vi "ActiveObjects_QueueQueue.vi"(7 "Action":T2=enum."GeneratePattern", 8 "error in (no error)":errorcluster, 10 "DataIn":variant, 11 "ClassRefToActOn":refnum<vi>) -> (0 "error out":errorcluster, 1 "Name":string, 2 "DataOut":variant, 3 "Cancelled":bool)   [LabVIEW 2020]
uses:
  <resource>/Framework/Providers/Open_GDS/ClassProviders/Provider_BaseClassInterface/BaseProvider_SubVIs/BaseProvider_DesignPatternsActions.ctl
  <resource>/Framework/Providers/Open_GDS/ClassProviders/Common/LvClass_class/GDSLvClass_ProviderTypes.ctl
  <resource>/Framework/Providers/Open_GDS/ClassProviders/Provider_EndevoGOOP400/EndevoG4ProviderName.ctl
  <resource>/Framework/Providers/Open_GDS/ClassProviders/Common/CommonVIs/CommonVIs_AttributeDataType.ctl
  <vilib>/picture/picture.llb/imagedata.ctl
  <resource>/Framework/Providers/Open_GDS/ClassProviders/Common/LvIcon_class/subvis/GDSLvIcon_TextDataType.ctl
  <resource>/Framework/Providers/Open_GDS/ClassProviders/Common/LvIcon_class/GDSLvIcon_WordCompressionType.ctl
  <resource>/Framework/Providers/Open_GDS/ClassProviders/Common/LvIcon_class/GDSLvIcon_TextAlignment.ctl
  <vilib>/Utility/lvfile.llb/NI_FileType.lvlib
panel:
  in  "ProcessCreation":T1(ring) caption="Process creation"
  out "NameExist1":string
  out "NameExist3":string
  out "NameExist2":string
  in  "AddInDestructor":bool
  in  "AddInConstructor":bool
  in  "StopName":string caption="Enter Stop Process Name"
  in  "StartName":string caption="Enter Start Process Name"
  in  "_Cancel":bool
  in  "_OK":bool
  in  "ProcessName":string caption="Enter Active Process Name"
  # "Active Object using Queues"
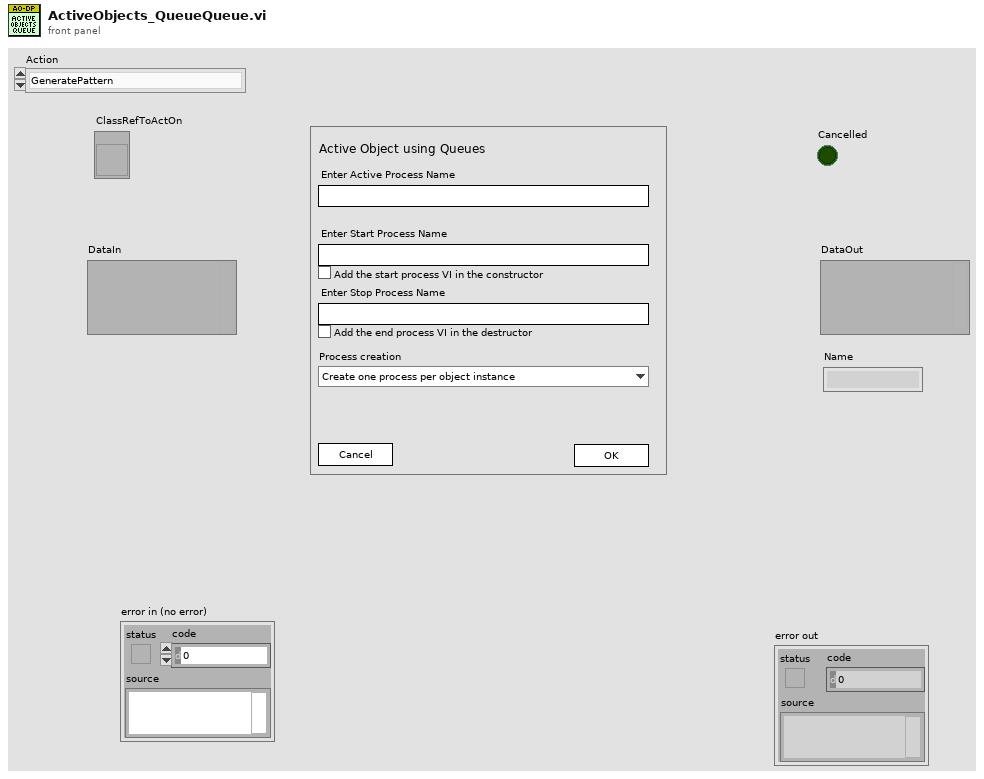
[diagram p1: front panel]
types:
  T1 = enum16{"Create one process per object instance", "Create only one process for this class"}
  T2 = typedef "BaseProvider_DesignPatternsActions.ctl" = enum16{"AddPatternDialog", "GeneratePattern", "RemovePattern", "CreatePatternMethod", "UpdatePattern"}
  T3 = typedef "GDSLvClass_ProviderTypes.ctl" = enum16{"UnKnown(LabVOOP)", "Native", "EndevoGOOP3", "OpenG(RootObject)", "OpenG(OpenG_Object)", "EndevoGOOP4", "JKI1"}
  T4 = cluster{"Data":cluster{"ProcessName":string, "StartName":string, "StopName":string, "AddInConstructor":bool, "AddInDestructor":bool, "ProcessCreation":enum16{"Create one process per object instance", "Create only one process for this class"}}, "ClassFolder":path, "SupportFolder":path, "ProcessCtl":refnum<vi>, "ProtectedFolder":refnum<vi>, "ProcessVI":refnum<vi>, "StartVI":refnum<vi>, "StopVI":refnum<vi>, "Application":refnum<vi>, "RepositoryVI":refnum<vi>, "ProcessIdRef":refnum<vi>, "ProcessRepository":path, "ClassProvider":T3, "TemplateName":string, "VI_ToFind":path, "MethodTemplate":path, "VI":refnum<vi>, "VI_ToFindSingleton":path, "Name":string}
  T5 = cluster{"ProcessName":string, "StartName":string, "StopName":string, "AddInConstructor":bool, "AddInDestructor":bool, "ProcessCreation":enum16{"Create one process per object instance", "Create only one process for this class"}}
  T6 = cluster{"Cancelled":bool, "Files":path[], "ClassPath":path, "DataOut":variant, "Name":string}
  T7 = enum8{"Enabled", "Disabled", "Disabled and Grayed Out"}
  T8 = typedef "EndevoG4ProviderName.ctl" = enum16{"EndevoGOOP400"}
  T9 = enum32{"invalid VI type", "Standard VI", "Control VI", "Global VI", "Polymorphic VI", "Configuration VI", "SubSystem", "Facade VI", "Method VI"}
  T10 = typedef "GDSLvIcon_TextDataType.ctl" = cluster{"Text":string, "Allow Only Capital Chars":bool, "Compression":T11, "Alignment":T12}
  T11 = typedef "GDSLvIcon_WordCompressionType.ctl" = enum16{"Auto", "On", "Off"}
  T12 = typedef "GDSLvIcon_TextAlignment.ctl" = enum16{"Center", "Left", "Right"}
  T13 = typedef "imagedata.ctl" = cluster{"image type":i32, "image depth":i32, "image":u8[], "mask":u8[], "colors":u32[], "Rectangle":cluster{"left":i16, "top":i16, "right":i16, "bottom":i16}}
  T14 = typedef "GDSLvCLass_ClassSettingsType.ctl" = cluster{"ClassProviderName":string, "ClassTemplateUsed":string, "ClassTemplateVersion":string, "ClassDescription":string, "PlugIns":T15[], "ConnectorPanePattern":string}
  T15 = typedef "GDSLvClass_PlugIn.ctl" = cluster{"Type":T16, "ID":string, "Version":string, "Path":path, "Name":string, "Data":variant}
  T16 = typedef "GDSLvClass_PlugInTypes.ctl" = enum16{"DesignPattern", "MethodTypes"}
  T17 = typedef "GOOP400_Options.ctl" = cluster{"FlatFolderStructure":bool}
  T18 = enum32{"invalid scope", "public", "private", "protected"}[]
  T19 = typedef "CommonVIs_AttributeDataType.ctl" = enum16{"UINT8", "INT8", "UINT16", "INT16", "UINT32", "INT32", "UINT64", "INT64", "SGL", "DBL", "EXT", "CSG", "CDB", "CXT", "TimeStamp", "STRING", "PATH", "BOOL", "ENUM", "RefNum", "VIRefNum", "LabVIEW Class", "Cluster", "Variant", "TypeDef", "Waveform", "LabVIEW Object", "Other", "void", "Set", "Map"}
  T20 = typedef "GDSLvClass_IconSettingsType.ctl" = cluster{"Frame":u32, "Frame thickness":u8, "Header Background":u32, "Header Text":u32, "ColorPublic":u32, "ColorProtected":u32, "ColorPrivate":u32, "Body Text":u32, "ClassBodyIcon":string}
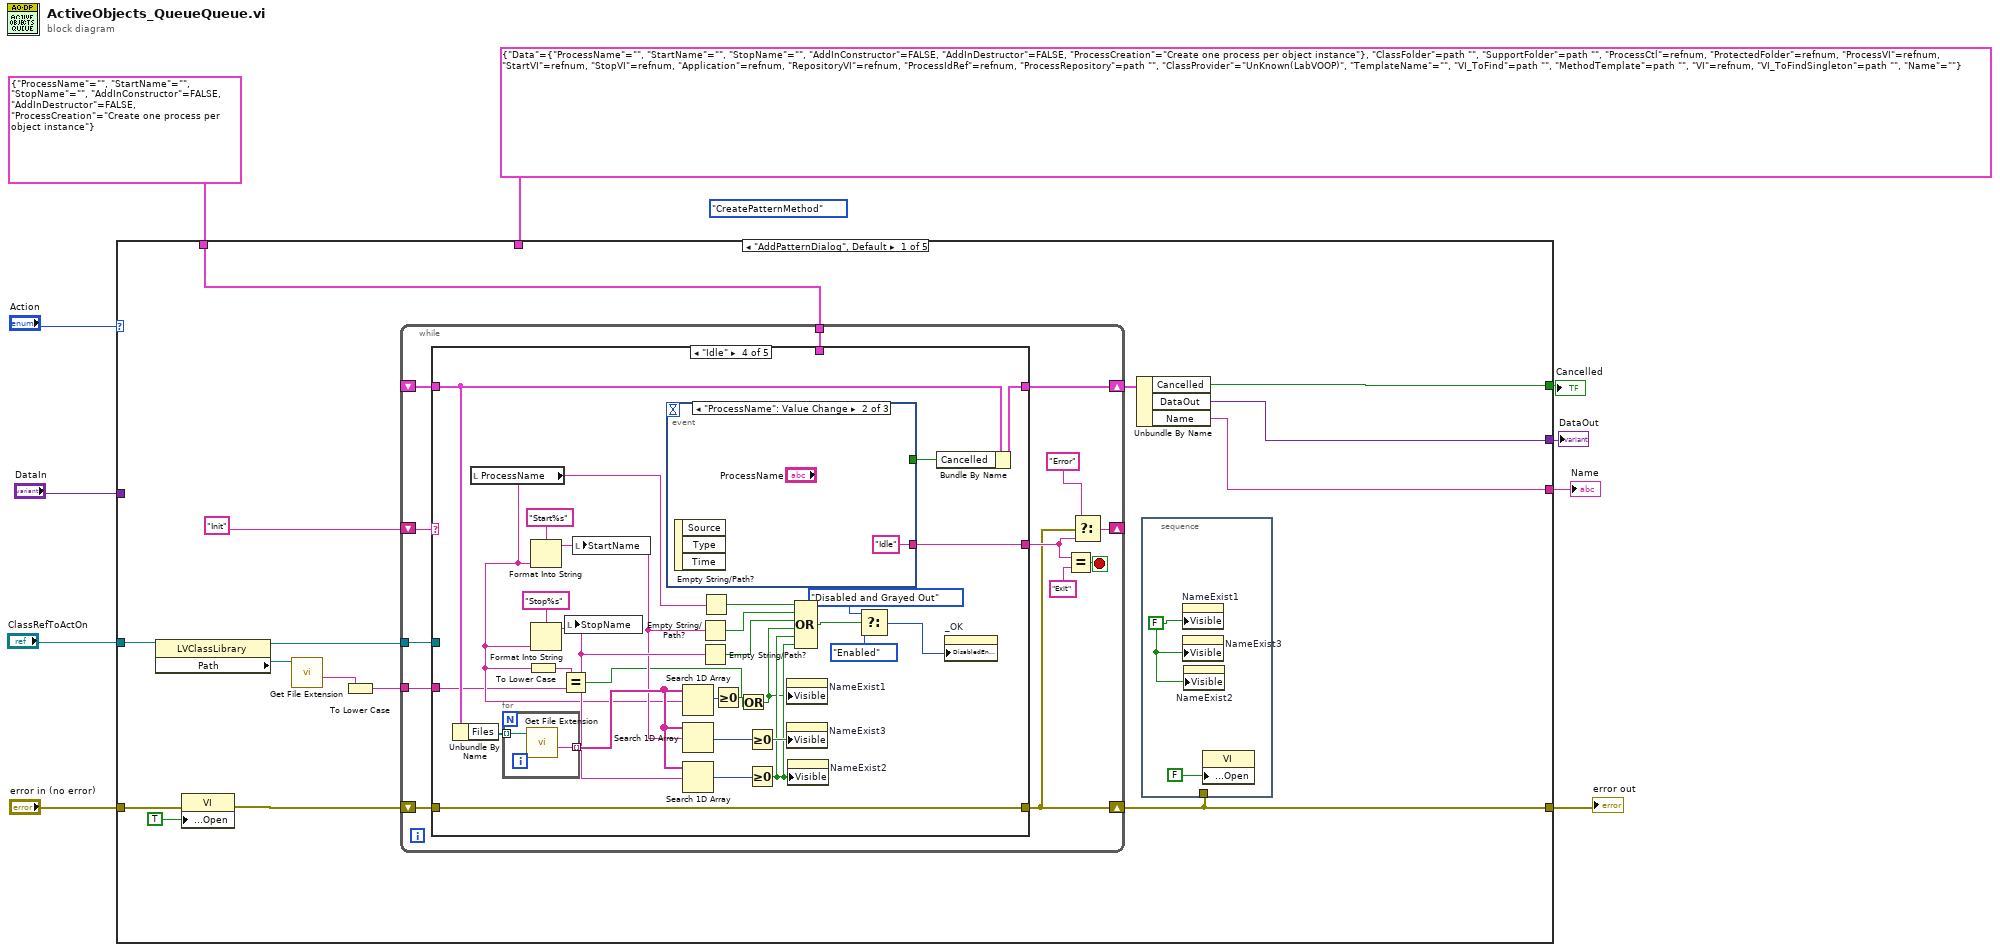
[diagram p0: block diagram]
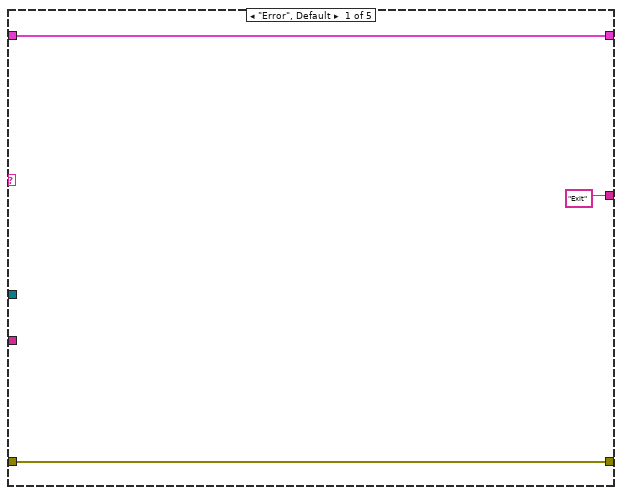
[diagram p2: hidden frame]
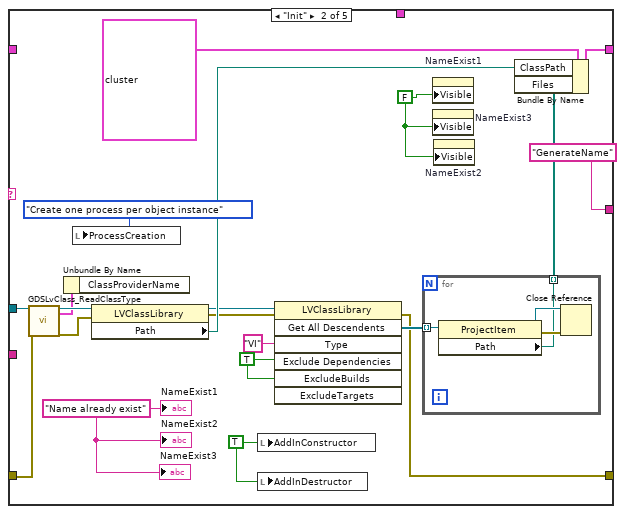
[diagram p3: hidden frame]
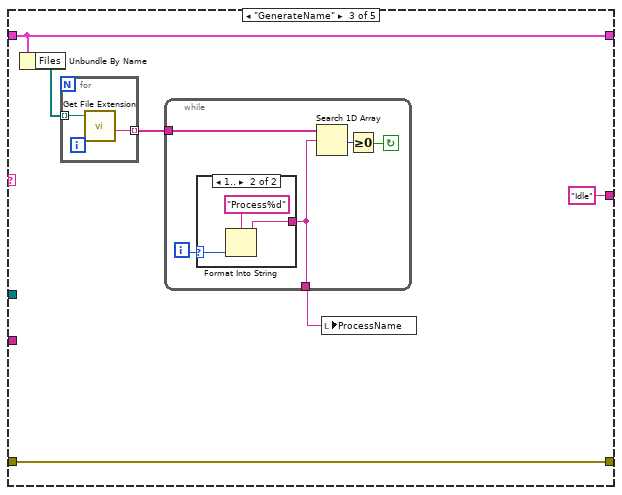
[diagram p4: hidden frame]
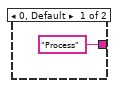
[diagram p5: hidden frame]
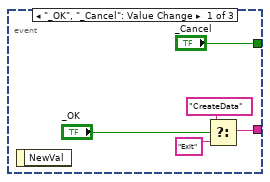
[diagram p6: hidden frame]
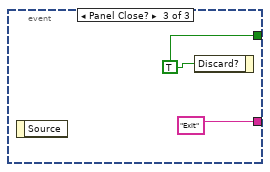
[diagram p7: hidden frame]
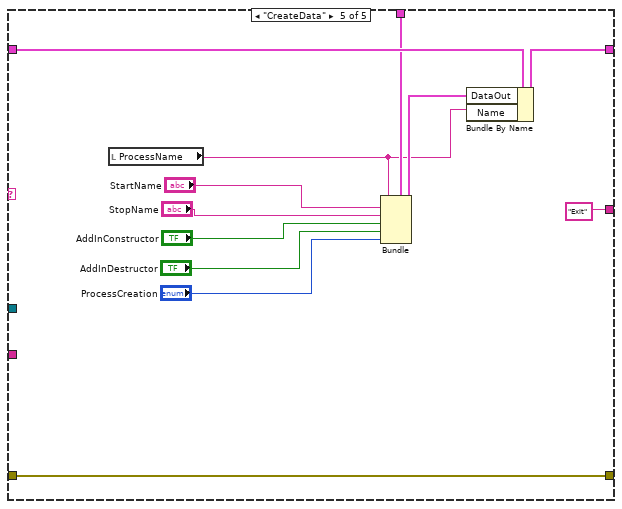
[diagram p8: hidden frame]
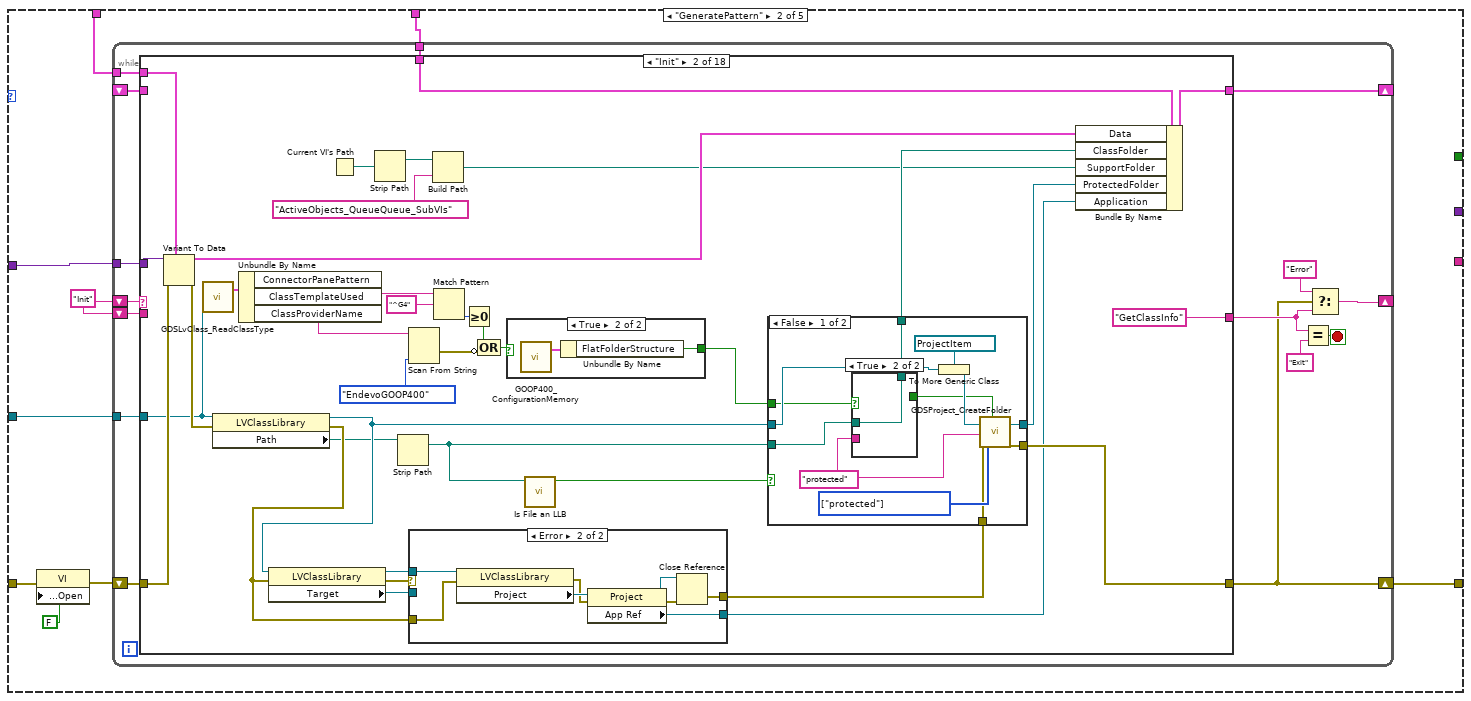
[diagram p9: hidden frame]
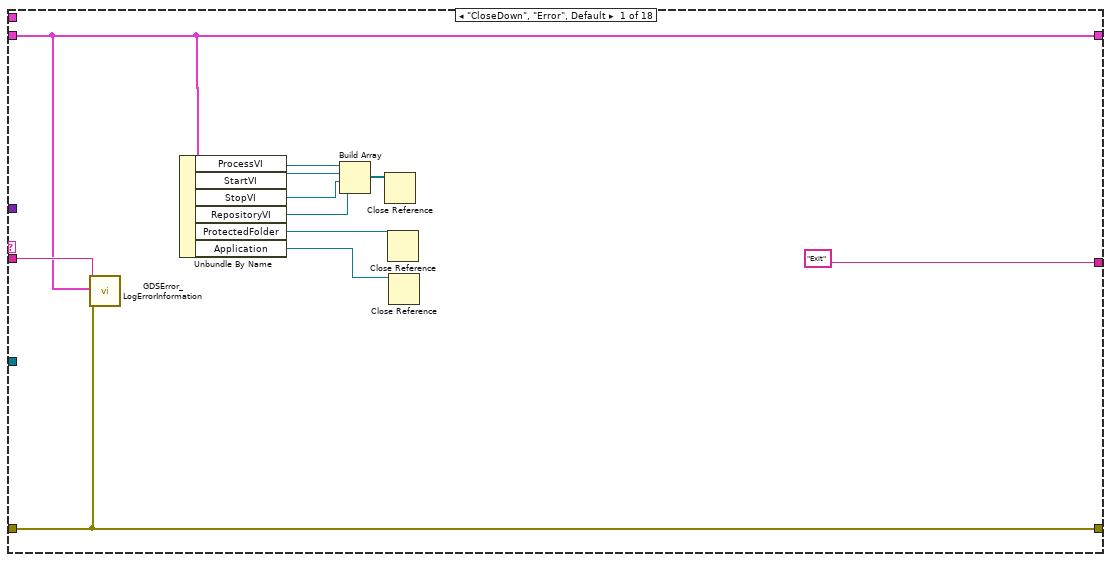
[diagram p10: hidden frame]
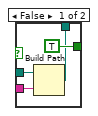
[diagram p12: hidden frame]
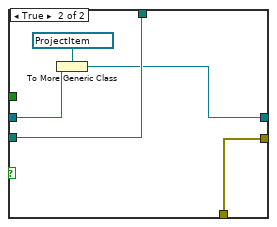
[diagram p13: hidden frame]
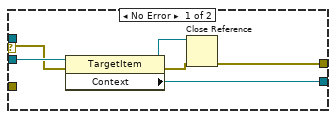
[diagram p14: hidden frame]
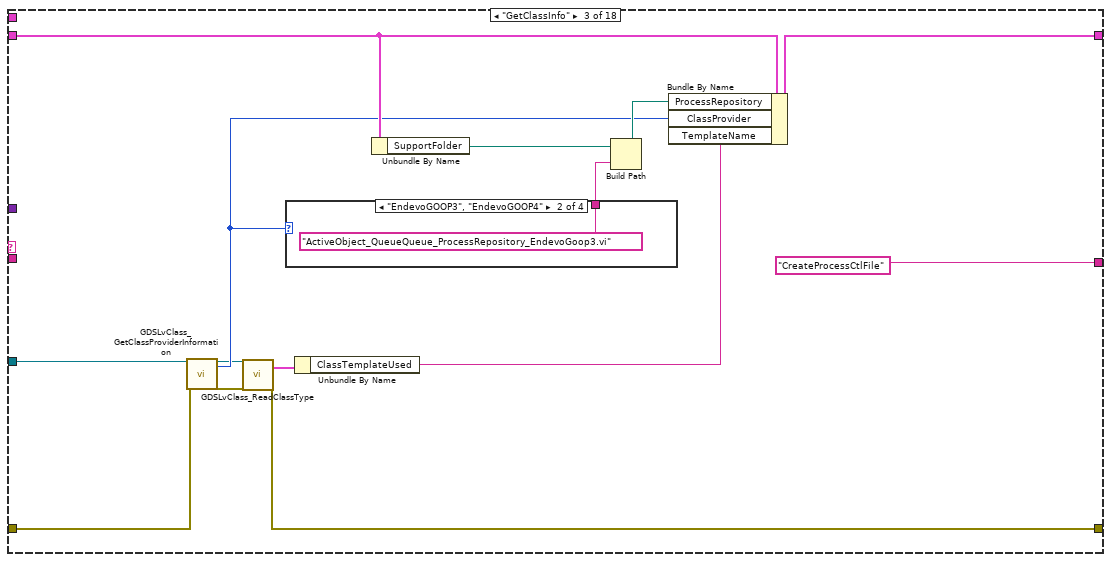
[diagram p15: hidden frame]
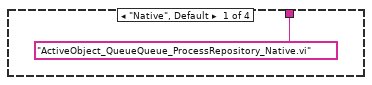
[diagram p16: hidden frame]
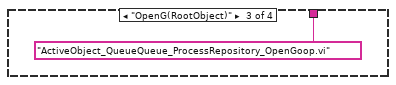
[diagram p17: hidden frame]
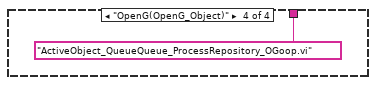
[diagram p18: hidden frame]
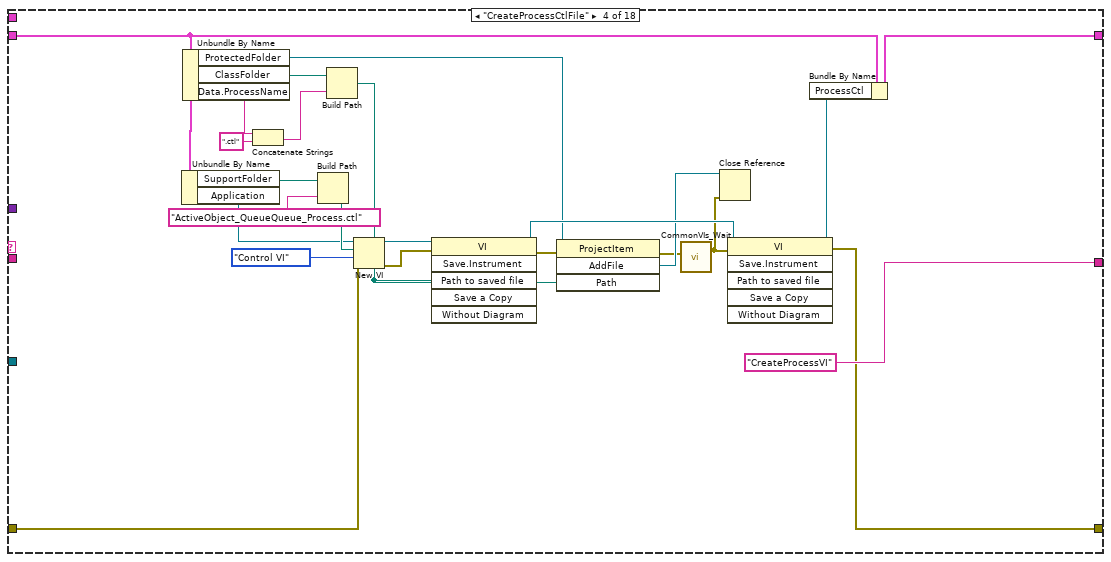
[diagram p19: hidden frame]
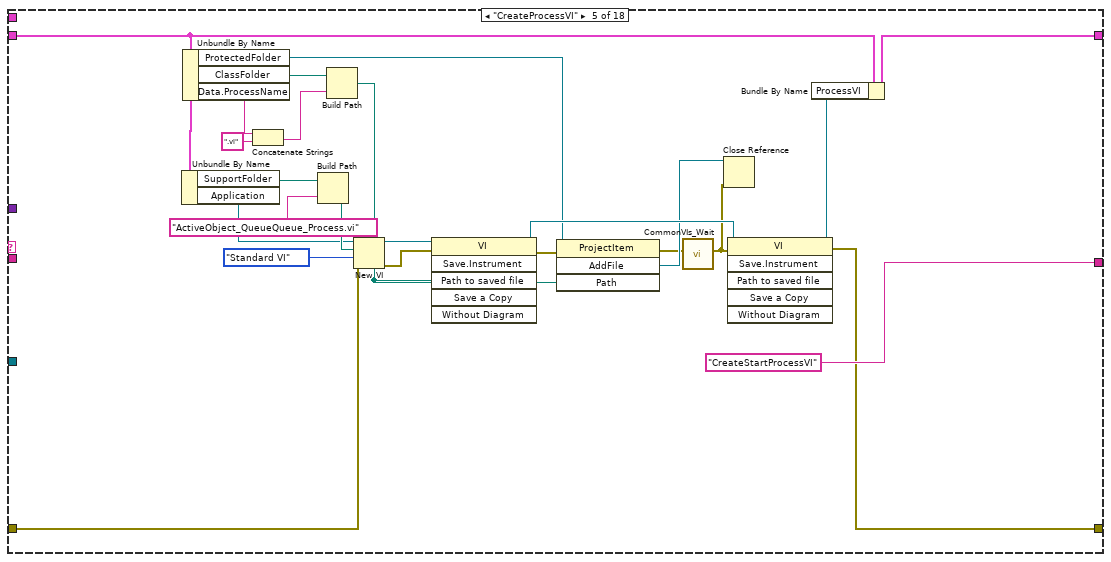
[diagram p20: hidden frame]
diagram:
  (unwired) BaseProvider_DesignPatternsActions."CreatePatternMethod" ("Action")
  n1 = case shown="\"AddPatternDialog\", Default" "Action" {
    tunnel: "error in (no error)" -> [w24 w138 w724 w725 w731]
    tunnel: [w21 w144 w724 w725 w726] -> w8
    tunnel: "ClassRefToActOn" -> [w14 w140 _ _ w730]
    tunnel: [w19 _ _ _ _] -> w6
    tunnel: [w18 _ _ _ _] -> w5
    tunnel: T5 {"ProcessName"="", "StartName"="", "StopName"="", "AddInConstructor"=FALSE, "AddInDestructor"=FALSE, "ProcessCreation"=enum."Create one process per object instance"} ("output cluster") -> [w17 w142 _ _ w727]
    tunnel: "DataIn" -> [_ w143 _ _ w729]
    tunnel: T4 {"Data"={"ProcessName"="", "StartName"="", "StopName"="", "AddInConstructor"=FALSE, "AddInDestructor"=FALSE, "ProcessCreation"=enum."Create one process per object instance"}, "ClassFolder"=path "", "SupportFolder"=path "", "ProcessCtl"=refnum, "ProtectedFolder"=refnum, "ProcessVI"=refnum, "StartVI"=refnum, "StopVI"=refnum, "Application"=refnum, "RepositoryVI"=refnum, "ProcessIdRef"=refnum, "ProcessRepository"=path "", "ClassProvider"=enum."UnKnown(LabVOOP)", "TemplateName"="", "VI_ToFind"=path "", "MethodTemplate"=path "", "VI"=refnum, "VI_ToFindSingleton"=path "", "Name"=""} -> [_ w141 _ _ w728]
    tunnel: [w16 _ _ _ _] -> w1
    frame "AddPatternDialog", Default {
      n2 = property class="LVClassLibrary"(reference=w14) -> (reference out=w13:refnum<vi>, "Path"=w15:path)  [unwired: 1 in, 1 out]
      n3 = property class="VI"(error in=w24, "Front Panel.Open"=TRUE ("Front Panel Window:Open")) -> (error out=w23:errorcluster)  [unwired: 1 in, 1 out]
      n4 = call <vilib>:"Get File Extension.vi"("file"=w15) -> ("filename without extension"=w11:string)  [unwired: 6 in, 4 out]
      n5 = To Lower Case(string=w11) -> (all lower case string=w12:string)
      n6 = while {
        shift-right: [w33] -> w21
        shift-left: w23 -> [w40]
        shift-right: [w38] -> _
        shift-left: "Init" -> [w39]
        shift-right: [w32] -> w20
        shift-left: _ -> [w31]
        tunnel: w13 -> [w30]
        tunnel: w17 -> [w29]
        tunnel: w12 -> [w28]
        stop <- w37 stop-if-true
        n7 = case shown="\"Idle\"" w39 {
          tunnel: w40 -> [w43 w47 w68 w112 w127]
          tunnel: [w43 w59 w68 w112 w127] -> w33
          tunnel: ["Exit" "GenerateName" "Idle" w113 "Exit"] -> w34
          tunnel: [w41 w57 w69 w111 w129] -> w32
          tunnel: w31 -> [w41 _ w69 w106 w131]
          tunnel: w30 -> [_ w49 _ _ _]
          tunnel: w29 -> [_ _ _ _ w126]
          tunnel: w28 -> [_ _ _ w87 _]
          frame "Error", Default {
          }
          frame "Init" {
            w50 = "Name already exist" ("NameExist1")
            w51 = FALSE ("Visible")
            w52 = TRUE ("AddInConstructor")
            w61 = TRUE ("ExcludeDependencies")
            n8 = call <resource>:"GDSLvClass_ReadClassType.vi"("Class Refnum In"=w49, "error in (no error)"=w47) -> ("Class Refnum Out"=w48:refnum<vi>, "ClassSettings"=w45:T14, "error out"=w46:errorcluster)  [unwired: 15 in]
            n9 = Unbundle By Name(w45) -> ()  [unwired: 1 out]
            n10 = local write "ProcessCreation"(T1."Create one process per object instance" ("ProcessCreation")) -> ()
            n11 = property class="LVClassLibrary"(reference=w48, error in=w46) -> (reference out=w54:refnum<vi>, error out=w53:errorcluster, "Path"=w56:path)
            n12 = local write "AddInConstructor"(w52) -> ()
            n13 = local write "AddInDestructor"(w52) -> ()
            n14 = invoke class="LVClassLibrary" method="Get All Descendents"(reference=w54, error in=w53, "Type"="VI", "Exclude Dependencies"=w61, "ExcludeBuilds"=w61) -> (error out=w59:errorcluster, "All Descendents"=w60:refnum<vi>[])  [unwired: 2 in, 5 out]
            n15 = for {
              tunnel: w60 -> [w67] mode=indexing
              tunnel: [w64] -> w55 mode=indexing
              n16 = property class="ProjectItem"(reference=w67) -> (reference out=w65:refnum<vi>, error out=w66:errorcluster, "Path"=w64:path)  [unwired: 1 in]
              n17 = Close Reference(reference=w65, error in (no error)=w66) -> ()  [unwired: 1 out]
            }
            n18 = property on="NameExist1" class="Str"("Visible"=w51) -> ()  [unwired: 2 in, 2 out]
            n19 = property on="NameExist3" class="Str"("Visible"=w51) -> ()  [unwired: 2 in, 2 out]
            n20 = property on="NameExist2" class="Str"("Visible"=w51) -> ()  [unwired: 2 in, 2 out]
            n21 = Bundle By Name(cluster=T6 {"Cancelled"=FALSE, "Files"=[], "ClassPath"=path "", "DataOut"=variant, "Name"=""}, "ClassPath"=w56, "Files"=w55) -> (w57:T6)
            "NameExist2" <- w50
            "NameExist3" <- w50
            "NameExist1" <- w50
          }
          frame "GenerateName" {
            n22 = Unbundle By Name(w69) -> ("Files"=w73:path[])
            n23 = for {
              tunnel: w73 -> [w84] mode=indexing
              tunnel: [w83] -> w72 mode=indexing
              n24 = call <vilib>:"Get File Extension.vi"("file"=w84) -> ("filename without extension"=w83:string)  [unwired: 6 in, 4 out]
            }
            n25 = while {
              tunnel: w72 -> [w77]
              tunnel: [w74] -> w71
              i -> [w78]
              stop <- w75 continue-if-true
              n26 = case shown="1.." w78 {
                selector: w78 -> [_ w81]
                tunnel: ["Process" ("format string") w80] -> w74
                frame 0, Default {
                }
                frame 1.. {
                  n27 = Format Into String(format string="Process%d", w81) -> (resulting string=w80:string)  [unwired: 2 in, 1 out]
                }
              }
              n28 = Search 1D Array(1D array=w77, element=w74) -> (index of element=w76:i32)  [unwired: 1 in]
              n29 = Greater Or Equal To 0?(x=w76) -> (x >= 0?=w75:bool)
            }
            n30 = local write "ProcessName"(w71) -> ()
          }
          frame "Idle" {
            n31 = Unbundle By Name(w106) -> ("Files"=w107:path[])
            n32 = local read "ProcessName"() -> (w88:string)
            n33 = for {
              tunnel: w107 -> [w115] mode=indexing
              tunnel: [w114] -> w105 mode=indexing
              n34 = call <vilib>:"Get File Extension.vi"("file"=w115) -> ("filename without extension"=w114:string)  [unwired: 6 in, 4 out]
            }
            n35 = To Lower Case(string=w88) -> (all lower case string=w89:string)
            n36 = Format Into String(format string="Start%s", w88) -> (resulting string=w98:string)  [unwired: 2 in, 1 out]
            n37 = Format Into String(format string="Stop%s", w88) -> (resulting string=w99:string)  [unwired: 2 in, 1 out]
            n38 = Equal?(x=w89, y=w87) -> (x = y?=w86:bool)
            n39 = local write "StopName"(w99) -> ()
            n40 = local write "StartName"(w98) -> ()
            n41 = event shown="[1] \"ProcessName\": Value Change" {
              selector: _ -> [_ _ _]
              dyn-events: _ -> [_ _ _]
              timeout: _ -> [_ _ _]
              tunnel: [w119 "Idle" "Exit"] -> w113
              tunnel: ["_Cancel" _ w122] -> w110
              event "_OK", "_Cancel": Value Change {
                n42 = event-data() -> ()  [unwired: 1 in, 1 out]
                n43 = Select(t="CreateData", s="_OK", f="Exit") -> (s? t:f=w119:string)
              }
              event "ProcessName": Value Change {
                n44 = event-data() -> ()  [unwired: 1 in, 3 out]
              }
              event Panel Close? {
                w122 = TRUE ("Discard?")
                n45 = event-data() -> ()  [unwired: 1 in, 1 out]
                n46 = event-data("Discard?"=w122) -> ()  [unwired: 1 in, 1 out]
              }
            }
            n47 = Search 1D Array(1D array=w105, element=w88) -> (index of element=w104:i32)  [unwired: 1 in]
            n48 = Search 1D Array(1D array=w105, element=w98) -> (index of element=w103:i32)  [unwired: 1 in]
            n49 = Search 1D Array(1D array=w105, element=w99) -> (index of element=w102:i32)  [unwired: 1 in]
            n50 = Empty String/Path?(string/path=w98) -> (empty?=w96:bool)
            n51 = Empty String/Path?(string/path=w99) -> (empty?=w97:bool)
            n52 = Empty String/Path?(string/path=w88) -> (empty?=w95:bool)
            n53 = Greater Or Equal To 0?(x=w104) -> (x >= 0?=w90:bool)
            n54 = Or(x=w86, y=w90) -> (x .or. y?=w85:bool)
            n55 = Greater Or Equal To 0?(x=w103) -> (x >= 0?=w101:bool)
            n56 = Greater Or Equal To 0?(x=w102) -> (x >= 0?=w100:bool)
            n57 = property on="NameExist1" class="Str"("Visible"=w85) -> ()  [unwired: 2 in, 2 out]
            n58 = property on="NameExist3" class="Str"("Visible"=w101) -> ()  [unwired: 2 in, 2 out]
            n59 = property on="NameExist2" class="Str"("Visible"=w100) -> ()  [unwired: 2 in, 2 out]
            n60 = Compound Arithmetic op=OR(w95, w96, w97, w85, w100, w100) -> (w94:bool)
            n61 = Select(t=T7."Disabled and Grayed Out" ("Disabled"), s=w94, f=T7."Enabled" ("Disabled")) -> (s? t:f=w91:T7)
            n62 = Bundle By Name(cluster=w106, "Cancelled"=w110) -> (w111:T6)
            n63 = property on="_OK" class="Bool"("DisabledEnum"=w91) -> ()  [unwired: 2 in, 2 out]
          }
          frame "CreateData" {
            n64 = local read "ProcessName"() -> (w124:string)
            n65 = Bundle(cluster=w126, "ProcessName"=w124, "StartName"="StartName", "StopName"="StopName", "AddInConstructor"="AddInConstructor", "AddInDestructor"="AddInDestructor", "ProcessCreation"="ProcessCreation") -> (w130:T5)
            n66 = Bundle By Name(cluster=w131, "DataOut"=w130, "Name"=w124) -> (w129:T6)
          }
        }
        n67 = Equal?(x=w34, y="Exit") -> (x = y?=w37:bool)
        n68 = Select(t="Error", s=w33, f=w34) -> (s? t:f=w38:string)
      }
      n69 = Unbundle By Name(w20) -> ("Cancelled"=w19:bool, "DataOut"=w18:variant, "Name"=w16:string)
      n70 = stacked-sequence {
        tunnel: w21 -> [_]
        frame #0 {
          w26 = FALSE ("Visible")
          n71 = property on="NameExist1" class="Str"("Visible"=w26) -> ()  [unwired: 2 in, 2 out]
          n72 = property on="NameExist3" class="Str"("Visible"=w26) -> ()  [unwired: 2 in, 2 out]
          n73 = property on="NameExist2" class="Str"("Visible"=w26) -> ()  [unwired: 2 in, 2 out]
          n74 = property class="VI"("Front Panel.Open"=FALSE ("Front Panel Window:Open")) -> ()  [unwired: 2 in, 2 out]
        }
      }
    }
    frame "GeneratePattern" {
      w136 = "Init"
      n75 = property class="VI"(error in=w138, "Front Panel.Open"=FALSE ("Front Panel Window:Open")) -> (error out=w137:errorcluster)  [unwired: 1 in, 1 out]
      n76 = while {
        shift-right: [w152] -> w144
        shift-left: w137 -> [w159]
        shift-right: [w157] -> _
        shift-left: w136 -> [w158]
        shift-right: [w151] -> _
        shift-left: _ -> [w150]
        tunnel: w143 -> [w149]
        tunnel: w142 -> [w148]
        tunnel: w141 -> [w147]
        tunnel: w140 -> [w146]
        shift-left: w136 -> [w145]
        stop <- w156 stop-if-true
        n77 = case shown="\"Init\"" w158 {
          tunnel: w159 -> [w162 w200 w256 w282 w306 w331 w357 w383 w399 w408 w437 w461 w484 w488 w544 w598 w651 w710]
          tunnel: [w162 w193 w247 w268 w292 w318 w344 w374 w389 w405 w420 w449 w475 w487 w543 w596 w649 w717] -> w152
          tunnel: ["Exit" "GetClassInfo" "CreateProcessCtlFile" "CreateProcessVI" "CreateStartProcessVI" "CreateStopProcessVI" "CreateProcessRepositoryVI" w367 "UpdateOORefInVIs" w404 "UpdateVIs" "UpdateRepositoryStaticVI" "FixViRefType" "UpdateIcons" "UpdateCreate?" "UpdateDestroy?" "SaveAll" "CloseDown"] -> w153
          tunnel: [w165 w205 w250 w271 w295 w321 w346 w376 w393 w412 w435 w441 w470 w489 w546 w594 w647 w712] -> w151
          tunnel: w150 -> [w165 _ w253 w272 w296 w322 w347 w365 w394 w412 w435 w441 w470 w489 w546 w594 w647 w712]
          tunnel: w149 -> [_ w204 _ _ _ _ _ _ _ _ _ _ _ _ _ _ _ _]
          tunnel: w148 -> [_ w203 _ _ _ _ _ _ _ _ _ _ _ _ _ _ _ _]
          tunnel: w147 -> [_ w202 _ _ _ _ _ _ _ _ _ _ _ _ _ _ _ _]
          tunnel: w146 -> [_ w174 w257 _ _ _ _ _ w391 w407 w426 _ _ _ w550 w593 w646 w716]
          tunnel: w145 -> [w169 _ _ _ _ _ _ _ _ _ _ _ _ _ _ _ _ _]
          frame "CloseDown", "Error", Default {
            n78 = call <resource>:"GDSError_LogErrorInformation.vi"("State"=w169, "LocalVariableData"=w165, "error in (no error)"=w162) -> ()  [unwired: 16 in, 1 out]
            n79 = Unbundle By Name(w165) -> ("ProcessVI"=w168:refnum<vi>, "StartVI"=w167:refnum<vi>, "StopVI"=w166:refnum<vi>, "RepositoryVI"=w164:refnum<vi>, "ProtectedFolder"=w161:refnum<vi>, "Application"=w160:refnum<vi>)
            n80 = Build Array(w168, w167, w166, w164) -> (w163:refnum<vi>[])
            n81 = Close Reference(reference=w163) -> ()  [unwired: 1 in, 1 out]
            n82 = Close Reference(reference=w161) -> ()  [unwired: 1 in, 1 out]
            n83 = Close Reference(reference=w160) -> ()  [unwired: 1 in, 1 out]
          }
          frame "Init" {
            n84 = Variant To Data(error in=w200, type=w203, Variant=w204) -> (data=w201:T5, error out=w194:errorcluster)
            n85 = call <resource>:"GDSLvClass_ReadClassType.vi"("Class Refnum In"=w174) -> ("ClassSettings"=w175:T14)  [unwired: 16 in, 2 out]
            n86 = property class="LVClassLibrary"(reference=w174, error in=w194) -> (reference out=w187:refnum<vi>, error out=w188:errorcluster, "Path"=w184:path)
            n87 = Unbundle By Name(w175) -> ("ClassTemplateUsed"=w173:string, "ClassProviderName"=w172:string)  [unwired: 1 out]
            n88 = property class="LVClassLibrary"(reference=w187, error in=w188) -> (reference out=w191:refnum<vi>, error out=w189:errorcluster, "Target"=w190:refnum<vi>)
            n89 = Current VI's Path() -> (path=w198:path)
            n90 = Strip Path(path=w198) -> (stripped path=w197:path)  [unwired: 1 out]
            n91 = Strip Path(path=w184) -> (stripped path=w182:path)  [unwired: 1 out]
            n92 = Scan From String(input string=w172, default 1=EndevoG4ProviderName."EndevoGOOP400" ("ProviderName")) -> (error out=w178:errorcluster)  [unwired: 4 in, 2 out]
            n93 = case shown="Error" w189 {
              selector: w189 -> [w232 _]
              tunnel: w190 -> [w236 _]
              tunnel: [w235 w238] -> w186
              tunnel: [w231 w239] -> w185
              tunnel: w191 -> [_ w244]
              tunnel: w188 -> [_ w243]
              frame No Error {
                n94 = property class="TargetItem"(reference=w236, error in=w232) -> (reference out=w233:refnum<vi>, error out=w234:errorcluster, "Context"=w235:refnum<vi>)
                n95 = Close Reference(reference=w233, error in (no error)=w234) -> (error out=w231:errorcluster)
              }
              frame Error {
                n96 = property class="LVClassLibrary"(reference=w244, error in=w243) -> (error out=w237:errorcluster, "Project"=w242:refnum<vi>)  [unwired: 1 out]
                n97 = property class="Project"(reference=w242, error in=w237) -> (reference out=w240:refnum<vi>, error out=w241:errorcluster, "App Ref"=w238:refnum<vi>)
                n98 = Close Reference(reference=w240, error in (no error)=w241) -> (error out=w239:errorcluster)
              }
            }
            n99 = Build Path(base path=w197, name or relative path="ActiveObjects_QueueQueue_SubVIs") -> (appended path=w195:path)
            n100 = Match Pattern(string=w173, regular expression="^G4") -> (offset past match=w179:i32)  [unwired: 1 in, 3 out]
            n101 = Greater Or Equal To 0?(x=w179) -> (x >= 0?=w177:bool)
            n102 = Compound Arithmetic op=OR(w177, invert w178) -> (w176:bool)
            n103 = case shown="True" w176 {
              tunnel: [_ w207] -> w171
              frame False {
              }
              frame True {
                n104 = call <resource>:"GOOP400_ConfigurationMemory.vi"() -> ("OptionsOut"=w208:T17)  [unwired: 18 in, 1 out]
                n105 = Unbundle By Name(w208) -> ("FlatFolderStructure"=w207:bool)
              }
            }
            n106 = call <vilib>:"Is File an LLB.vi"("path"=w182) -> ("Is LLB?"=w183:bool)  [unwired: 9 in, 1 out]
            n107 = case shown="False" w183 {
              tunnel: [w215 w227] -> w199
              tunnel: [w214 w228] -> w193
              tunnel: [w213 w226] -> w192
              tunnel: w187 -> [w212 w229]
              tunnel: w185 -> [w211 w228]
              tunnel: w182 -> [w210 w227]
              tunnel: w171 -> [w209 _]
              frame False {
                w218 = T18 [enum."protected"] items=["invalid scope", "public", "private", "protected"] ("FolderScope")
                w217 = "protected" ("name or relative path")
                n108 = case shown="True" w209 {
                  tunnel: w217 -> [w224 _]
                  tunnel: [TRUE ("CreateThePhysicalFolderIfPossible(False)") _] -> w216
                  tunnel: [w222 w225] -> w215
                  tunnel: w210 -> [w221 w225]
                  frame False {
                    n109 = Build Path(base path=w221, name or relative path=w224) -> (appended path=w222:path)
                  }
                  frame True {
                  }
                }
                n110 = To More Generic Class(target class=refnum<vi> refnum ("AddItem"), reference=w212) -> (generic class reference=w219:refnum<vi>)
                n111 = call <resource>:"GDSProject_CreateFolder.vi"("Project Item To Create Folder Below(Use MyComputer if not wired)"=w219, "FolderName"=w217, "error in (no error)"=w211, "FolderScope"=w218, "CreateThePhysicalFolderIfPossible(False)"=w216) -> ("ItemOut"=w213:refnum<vi>, "error out"=w214:errorcluster)  [unwired: 11 in, 2 out]
              }
              frame True {
                n112 = To More Generic Class(target class=refnum<vi> refnum ("AddItem"), reference=w229) -> (generic class reference=w226:refnum<vi>)
              }
            }
            n113 = Bundle By Name(cluster=w202, "Data"=w201, "ClassFolder"=w199, "SupportFolder"=w195, "ProtectedFolder"=w192, "Application"=w186) -> (w205:T4)
          }
          frame "GetClassInfo" {
            n114 = call <resource>:"GDSLvClass_GetClassProviderInformation.vi"("Class Refnum In"=w257, "error in (no error)"=w256) -> ("Class Refnum Out"=w249:refnum<vi>, "ClassProvider"=w251:T3, "error out"=w248:errorcluster)  [unwired: 15 in]
            n115 = call <resource>:"GDSLvClass_ReadClassType.vi"("Class Refnum In"=w249, "error in (no error)"=w248) -> ("ClassSettings"=w246:T14, "error out"=w247:errorcluster)  [unwired: 15 in, 1 out]
            n116 = case shown="\"EndevoGOOP3\", \"EndevoGOOP4\"" w251 {
              tunnel: ["ActiveObject_QueueQueue_ProcessRepository_Native.vi" ("name or relative path") "ActiveObject_QueueQueue_ProcessRepository_EndevoGoop3.vi" ("name or relative path") "ActiveObject_QueueQueue_ProcessRepository_OpenGoop.vi" ("name or relative path") "ActiveObject_QueueQueue_ProcessRepository_OGoop.vi" ("name or relative path")] -> w254
              frame "Native", Default {
              }
              frame "EndevoGOOP3", "EndevoGOOP4" {
              }
              frame "OpenG(RootObject)" {
              }
              frame "OpenG(OpenG_Object)" {
              }
            }
            n117 = Unbundle By Name(w246) -> ("ClassTemplateUsed"=w245:string)
            n118 = Unbundle By Name(w253) -> ("SupportFolder"=w255:path)
            n119 = Build Path(base path=w255, name or relative path=w254) -> (appended path=w252:path)
            n120 = Bundle By Name(cluster=w253, "ProcessRepository"=w252, "ClassProvider"=w251, "TemplateName"=w245) -> (w250:T4)
          }
          frame "CreateProcessCtlFile" {
            n121 = Unbundle By Name(w272) -> ("SupportFolder"=w278:path, "Application"=w266:refnum<vi>)
            n122 = Unbundle By Name(w272) -> ("ProtectedFolder"=w267:refnum<vi>, "ClassFolder"=w286:path, "Data.ProcessName"=w285:string)
            n123 = Concatenate Strings(w285, ".ctl" ("string")) -> (w283:string)
            n124 = Build Path(base path=w278, name or relative path="ActiveObject_QueueQueue_Process.ctl") -> (appended path=w276:path)
            n125 = Build Path(base path=w286, name or relative path=w283) -> (appended path=w274:path)
            n126 = New VI(8:w282, 9:T9."Control VI" ("vi type (standard vi)"), 10:w276, 11:w266) -> (0:w279:errorcluster, 3:w280:refnum<vi>)  [unwired: 3 in]
            n127 = invoke class="VI" method="Save.Instrument"(reference=w280, error in=w279, "Path to saved file"=w274) -> (reference out=w273:refnum<vi>, error out=w275:errorcluster)  [unwired: 3 in, 4 out]
            n128 = invoke class="ProjectItem" method="AddFile"(reference=w267, error in=w275, "Path"=w274) -> (error out=w264:errorcluster, "AddFile"=w265:refnum<vi>)  [unwired: 1 in, 2 out]
            n129 = call <resource>:"CommonVIs_Wait.vi"("error in"=w264) -> ("error out"=w263:errorcluster)  [unwired: 9 in]
            n130 = Close Reference(reference=w265, error in (no error)=w263) -> ()  [unwired: 1 out]
            n131 = invoke class="VI" method="Save.Instrument"(reference=w273, error in=w263) -> (reference out=w270:refnum<vi>, error out=w268:errorcluster)  [unwired: 4 in, 4 out]
            n132 = Bundle By Name(cluster=w272, "ProcessCtl"=w270) -> (w271:T4)
          }
          frame "CreateProcessVI" {
            n133 = Unbundle By Name(w296) -> ("SupportFolder"=w302:path, "Application"=w290:refnum<vi>)
            n134 = Unbundle By Name(w296) -> ("ProtectedFolder"=w291:refnum<vi>, "ClassFolder"=w310:path, "Data.ProcessName"=w309:string)
            n135 = Concatenate Strings(w309, ".vi" ("string")) -> (w307:string)
            n136 = Build Path(base path=w302, name or relative path="ActiveObject_QueueQueue_Process.vi") -> (appended path=w300:path)
            n137 = Build Path(base path=w310, name or relative path=w307) -> (appended path=w298:path)
            n138 = New VI(8:w306, 9:T9."Standard VI" ("vi type (standard vi)"), 10:w300, 11:w290) -> (0:w303:errorcluster, 3:w304:refnum<vi>)  [unwired: 3 in]
            n139 = invoke class="VI" method="Save.Instrument"(reference=w304, error in=w303, "Path to saved file"=w298) -> (reference out=w297:refnum<vi>, error out=w299:errorcluster)  [unwired: 3 in, 4 out]
            n140 = invoke class="ProjectItem" method="AddFile"(reference=w291, error in=w299, "Path"=w298) -> (error out=w288:errorcluster, "AddFile"=w289:refnum<vi>)  [unwired: 1 in, 2 out]
            n141 = call <resource>:"CommonVIs_Wait.vi"("error in"=w288) -> ("error out"=w287:errorcluster)  [unwired: 9 in]
            n142 = Close Reference(reference=w289, error in (no error)=w287) -> ()  [unwired: 1 out]
            n143 = invoke class="VI" method="Save.Instrument"(reference=w297, error in=w287) -> (reference out=w294:refnum<vi>, error out=w292:errorcluster)  [unwired: 4 in, 4 out]
            n144 = Bundle By Name(cluster=w296, "ProcessVI"=w294) -> (w295:T4)
          }
          frame "CreateStartProcessVI" {
            n145 = Unbundle By Name(w322) -> ("SupportFolder"=w327:path, "Application"=w316:refnum<vi>, "Data.ProcessCreation"=w315:T1)
            n146 = Unbundle By Name(w322) -> ("ProtectedFolder"=w317:refnum<vi>, "ClassFolder"=w335:path, "Data.StartName"=w334:string)
            n147 = case shown="\"Create one process per object instance\", Default" w315 {
              tunnel: ["ActiveObject_QueueQueue_StartProcess_OnePerObject.vi" ("name or relative path") "ActiveObject_QueueQueue_StartProcess_OnePerClass.vi" ("name or relative path")] -> w314
              frame "Create one process per object instance", Default {
              }
              frame "Create only one process for this class" {
              }
            }
            n148 = Concatenate Strings(w334, ".vi" ("string")) -> (w332:string)
            n149 = Build Path(base path=w327, name or relative path=w314) -> (appended path=w326:path)
            n150 = Build Path(base path=w335, name or relative path=w332) -> (appended path=w324:path)
            n151 = New VI(8:w331, 9:T9."Standard VI" ("vi type (standard vi)"), 10:w326, 11:w316) -> (0:w328:errorcluster, 3:w329:refnum<vi>)  [unwired: 3 in]
            n152 = invoke class="VI" method="Save.Instrument"(reference=w329, error in=w328, "Path to saved file"=w324) -> (reference out=w323:refnum<vi>, error out=w325:errorcluster)  [unwired: 3 in, 4 out]
            n153 = invoke class="ProjectItem" method="AddFile"(reference=w317, error in=w325, "Path"=w324) -> (error out=w312:errorcluster, "AddFile"=w313:refnum<vi>)  [unwired: 1 in, 2 out]
            n154 = call <resource>:"CommonVIs_Wait.vi"("error in"=w312) -> ("error out"=w311:errorcluster)  [unwired: 9 in]
            n155 = Close Reference(reference=w313, error in (no error)=w311) -> ()  [unwired: 1 out]
            n156 = invoke class="VI" method="Save.Instrument"(reference=w323, error in=w311) -> (reference out=w320:refnum<vi>, error out=w318:errorcluster)  [unwired: 4 in, 4 out]
            n157 = Bundle By Name(cluster=w322, "StartVI"=w320) -> (w321:T4)
          }
          frame "CreateStopProcessVI" {
            n158 = Unbundle By Name(w347) -> ("SupportFolder"=w353:path, "Application"=w342:refnum<vi>)
            n159 = Unbundle By Name(w347) -> ("ProtectedFolder"=w343:refnum<vi>, "ClassFolder"=w361:path, "Data.StopName"=w360:string)
            n160 = Concatenate Strings(w360, ".vi" ("string")) -> (w358:string)
            n161 = Build Path(base path=w353, name or relative path="ActiveObject_QueueQueue_StopProcess.vi") -> (appended path=w351:path)
            n162 = Build Path(base path=w361, name or relative path=w358) -> (appended path=w349:path)
            n163 = New VI(8:w357, 9:T9."Standard VI" ("vi type (standard vi)"), 10:w351, 11:w342) -> (0:w354:errorcluster, 3:w355:refnum<vi>)  [unwired: 3 in]
            n164 = invoke class="VI" method="Save.Instrument"(reference=w355, error in=w354, "Path to saved file"=w349) -> (reference out=w348:refnum<vi>, error out=w350:errorcluster)  [unwired: 3 in, 4 out]
            n165 = invoke class="ProjectItem" method="AddFile"(reference=w343, error in=w350, "Path"=w349) -> (error out=w339:errorcluster, "AddFile"=w340:refnum<vi>)  [unwired: 1 in, 2 out]
            n166 = call <resource>:"CommonVIs_Wait.vi"("error in"=w339) -> ("error out"=w338:errorcluster)  [unwired: 9 in]
            n167 = Close Reference(reference=w340, error in (no error)=w338) -> ()  [unwired: 1 out]
            n168 = invoke class="VI" method="Save.Instrument"(reference=w348, error in=w338) -> (reference out=w345:refnum<vi>, error out=w344:errorcluster)  [unwired: 4 in, 4 out]
            n169 = Bundle By Name(cluster=w347, "StopVI"=w345) -> (w346:T4)
          }
          frame "CreateProcessRepositoryVI" {
            n170 = Unbundle By Name(w365) -> ("ClassProvider"=w364:T3)
            n171 = Unbundle By Name(w365) -> ("ProcessRepository"=w366:path, "Application"=w372:refnum<vi>)
            n172 = Unbundle By Name(w365) -> ("ProtectedFolder"=w373:refnum<vi>, "ClassFolder"=w384:path, "Data.ProcessName"=w371:string)
            n173 = Format Into String(format string="%sRepository.vi", w371) -> (resulting string=w369:string)  [unwired: 2 in, 1 out]
            n174 = New VI(8:w383, 9:T9."Standard VI" ("vi type (standard vi)"), 10:w366, 11:w372) -> (0:w380:errorcluster, 3:w381:refnum<vi>)  [unwired: 3 in]
            n175 = Build Path(base path=w384, name or relative path=w369) -> (appended path=w378:path)
            n176 = invoke class="VI" method="Save.Instrument"(reference=w381, error in=w380, "Path to saved file"=w378) -> (reference out=w377:refnum<vi>, error out=w379:errorcluster)  [unwired: 3 in, 4 out]
            n177 = invoke class="ProjectItem" method="AddFile"(reference=w373, error in=w379, "Path"=w378) -> (error out=w363:errorcluster, "AddFile"=w368:refnum<vi>)  [unwired: 1 in, 2 out]
            n178 = case shown="Default" w364 {
              tunnel: ["UpdateOORefInVIs" "AddCtlToAttribute"] -> w367
              frame Default {
              }
              frame "UnKnown(LabVOOP)", "Native" {
              }
            }
            n179 = call <resource>:"CommonVIs_Wait.vi"("error in"=w363) -> ("error out"=w362:errorcluster)  [unwired: 9 in]
            n180 = Close Reference(reference=w368, error in (no error)=w362) -> ()  [unwired: 1 out]
            n181 = invoke class="VI" method="Save.Instrument"(reference=w377, error in=w362) -> (reference out=w375:refnum<vi>, error out=w374:errorcluster)  [unwired: 4 in, 4 out]
            n182 = Bundle By Name(cluster=w365, "RepositoryVI"=w375) -> (w376:T4)
          }
          frame "AddCtlToAttribute" {
            w387 = T19[] [enum."UINT32"] items=["UINT8", "INT8", "UINT16", "INT16", "UINT32", "INT32", "UINT64", "INT64", "SGL", "DBL", "EXT", "CSG", "CDB", "CXT", "TimeStamp", "STRING", "PATH", "BOOL", "ENUM", "RefNum", "VIRefNum", "LabVIEW Class", "Cluster", "Variant", "TypeDef", "Waveform", "LabVIEW Object", "Other", "void", "Set", "Map"] ("DataTypes")
            n183 = call <resource>:"Scripting_PlaceControlsInClassAttribute.vi"("ClassRefnum"=w391, "DeleteAllCurrentAttributesFirst(True)"=FALSE, "ControlNames"=string[] ["ProcessId:Process#No"], "DataTypes"=w387, "error in"=w399, "DeleteReferencesToCreatedAttributes(True)"=FALSE) -> ("ControlsCreated"=w395:refnum<vi>[], "error out"=w390:errorcluster)  [unwired: 7 in, 1 out]
            n184 = Index Array(array=w395) -> (element=w392:refnum<vi>)  [unwired: 1 in]
            n185 = call <resource>:"GDSLvClass_SaveEverythingInClass.vi"("ClassRefIn"=w391, "error in"=w390) -> ("error out"=w389:errorcluster)  [unwired: 16 in, 1 out]
            n186 = Bundle By Name(cluster=w394, "ProcessIdRef"=w392) -> (w393:T4)
          }
          frame "UpdateOORefInVIs" {
            n187 = property class="LVClassLibrary"(reference=w407) -> ("Path"=w403:path)  [unwired: 1 in, 2 out]
            n188 = Unbundle By Name(w412) -> ("ProcessVI"=w411:refnum<vi>, "StartVI"=w410:refnum<vi>, "StopVI"=w409:refnum<vi>, "RepositoryVI"=w401:refnum<vi>, "ClassProvider"=w400:T3)
            n189 = Build Array(w411, w410, w409, w401) -> (w406:refnum<vi>[])
            n190 = Path To String(path=w403) -> (string=w402:string)
            n191 = for {
              tunnel: w406 -> [w415] mode=indexing
              shift-right: [w418] -> w405
              shift-left: w408 -> [w417]
              tunnel: w402 -> [w416]
              n192 = call <resource>:"Scripting_ReplaceOORef.vi"("ViRef"=w415, "NewLvClassFile(ProjectPath or LvClassPath)"=w416, "error in (no error)"=w417) -> ("error out"=w418:errorcluster)  [unwired: 16 in]
            }
            n193 = case shown="Default" w400 {
              tunnel: ["UpdateVIs" "RenameProcessIdControl"] -> w404
              frame Default {
              }
              frame "UnKnown(LabVOOP)", "Native" {
              }
            }
          }
          frame "RenameProcessIdControl" {
            w419 = T19[] [enum."UINT32"] items=["UINT8", "INT8", "UINT16", "INT16", "UINT32", "INT32", "UINT64", "INT64", "SGL", "DBL", "EXT", "CSG", "CDB", "CXT", "TimeStamp", "STRING", "PATH", "BOOL", "ENUM", "RefNum", "VIRefNum", "LabVIEW Class", "Cluster", "Variant", "TypeDef", "Waveform", "LabVIEW Object", "Other", "void", "Set", "Map"] ("DataTypes")
            n194 = Unbundle By Name(w435) -> ("ProcessIdRef"=w438:refnum<vi>, "Data.ProcessName"=w433:string)
            n195 = Format Into String(format string="ProcessId:%s", w433) -> (resulting string=w432:string)  [unwired: 2 in, 1 out]
            n196 = property class="Ctl"(reference=w438, error in=w437, "Label.Text"=w432) -> (error out=w428:errorcluster)  [unwired: 1 out]
            n197 = call <resource>:"Scripting_PlaceControlsInClassAttribute.vi"("ClassRefnum"=w426, "DeleteAllCurrentAttributesFirst(True)"=FALSE, "ControlNames"=string[] ["DummyStringThatShouldBeDeleted"], "DataTypes"=w419, "error in"=w428, "DeleteReferencesToCreatedAttributes(True)"=FALSE) -> ("ControlsCreated"=w425:refnum<vi>[], "error out"=w427:errorcluster)  [unwired: 7 in, 1 out]
            n198 = Index Array(array=w425) -> (element=w424:refnum<vi>)  [unwired: 1 in]
            n199 = call <resource>:"GDSLvClass_SaveEverythingInClass.vi"("ClassRefIn"=w426, "ForceResaving(False)"=TRUE, "error in"=w427) -> ("ClassRefOut"=w422:refnum<vi>, "error out"=w421:errorcluster)  [unwired: 15 in]
            n200 = invoke class="Ctl" method="Delete"(reference=w424, error in=w421) -> (error out=w423:errorcluster)  [unwired: 1 in, 2 out]
            n201 = call <resource>:"GDSLvClass_SaveEverythingInClass.vi"("ClassRefIn"=w422, "error in"=w423) -> ("error out"=w420:errorcluster)  [unwired: 16 in, 1 out]
          }
          frame "UpdateVIs" {
            n202 = Unbundle By Name(w441) -> ("ProcessVI"=w453:refnum<vi>, "StartVI"=w452:refnum<vi>, "StopVI"=w451:refnum<vi>, "RepositoryVI"=w447:refnum<vi>)
            n203 = Unbundle By Name(w441) -> ("SupportFolder"=w443:path)
            n204 = Unbundle By Name(w441) -> ("RepositoryVI"=w462:refnum<vi>, "ProcessCtl"=w456:refnum<vi>)
            n205 = Unbundle By Name(w441) -> ("SupportFolder"=w460:path)
            n206 = Build Array(w453, w452, w451) -> (w448:refnum<vi>[])
            n207 = property class="VI"(reference=w447) -> ("Path"=w446:path)  [unwired: 1 in, 2 out]
            n208 = Build Path(base path=w443, name or relative path="ActiveObject_QueueQueue_ProcessRepository_Native.vi") -> (appended path=w440:path)
            n209 = property class="VI"(reference=w456) -> ("Path"=w455:path)  [unwired: 1 in, 2 out]
            n210 = Build Path(base path=w460, name or relative path="ActiveObject_QueueQueue_Process.ctl") -> (appended path=w458:path)
            n211 = Build Array(w446) -> (w445:path[])
            n212 = Build Array(w458) -> (w457:path[])
            n213 = Build Array(w455) -> (w454:path[])
            n214 = Build Array(w440) -> (w444:path[])
            n215 = call <resource>:"Scripting_ReplaceVisAndControls.vi"("ViRef"=w462, "OldVIsAndControls"=w457, "NewVIsAndControls"=w454, "error in (no error)"=w461) -> ("error out"=w450:errorcluster)  [unwired: 14 in, 1 out]
            n216 = for {
              shift-right: [w467] -> w449
              shift-left: w450 -> [w468]
              tunnel: w448 -> [w466] mode=indexing
              tunnel: w445 -> [w465]
              tunnel: w444 -> [w464]
              n217 = call <resource>:"Scripting_ReplaceVisAndControls.vi"("ViRef"=w466, "OldVIsAndControls"=w464, "NewVIsAndControls"=w465, "error in (no error)"=w468) -> ("error out"=w467:errorcluster)  [unwired: 14 in, 1 out]
            }
          }
          frame "UpdateRepositoryStaticVI" {
            w481 = refnum<vi> refnum  # StaticVIReference
            n218 = Unbundle By Name(w470) -> ("RepositoryVI"=w485:refnum<vi>)
            n219 = Unbundle By Name(w470) -> ("ClassFolder"=w474:path, "Data.ProcessName"=w473:string)
            n220 = Concatenate Strings(w473, ".vi" ("string")) -> (w471:string)
            n221 = Build Path(base path=w474, name or relative path=w471) -> (appended path=w469:path)
            n222 = call <resource>:"Scripting_FindNodeOnDiagram.vi"("ViRef(Ignored If Not Wired)"=w485, "NodeTypesToSearchFor"=string[] ["StaticVIReference"], "error in (no error)"=w484) -> ("Nodes"=w477:refnum<vi>[], "error out"=w476:errorcluster)  [unwired: 15 in]
            n223 = Index Array(array=w477) -> (element=w482:refnum<vi>)  [unwired: 1 in]
            n224 = To More Specific Class(target class=w481, reference=w482, error in=w476) -> (specific class reference=w480:refnum<vi>, error out=w479:errorcluster)
            n225 = property class="StatVIRef"(reference=w480, error in=w479, "Path"=w469) -> (error out=w478:errorcluster)  [unwired: 1 out]
            n226 = Close Reference(reference=w477, error in (no error)=w478) -> (error out=w475:errorcluster)
          }
          frame "FixViRefType" {
            w515 = refnum<vi> refnum  # VIRefNum
            w500 = refnum<vi> refnum  # VIRefNum
            w492 = refnum<vi> refnum  # Cluster
            n227 = Unbundle By Name(w489) -> ("ProcessCtl"=w525:refnum<vi>, "RepositoryVI"=w526:refnum<vi>, "ProcessVI"=w517:refnum<vi>)
            n228 = property class="VI"(reference=w525, error in=w488) -> (reference out=w504:refnum<vi>, error out=w494:errorcluster, "Panel"=w490:refnum<vi>)
            n229 = property class="Pnl"(reference=w490, error in=w494) -> (reference out=w505:refnum<vi>, error out=w493:errorcluster, "Controls[]"=w506:refnum<vi>[])
            n230 = Index Array(array=w506) -> (element=w491:refnum<vi>)  [unwired: 1 in]
            n231 = To More Specific Class(target class=w492, reference=w491, error in=w493) -> (specific class reference=w495:refnum<vi>, error out=w496:errorcluster)
            n232 = property class="Clust"(reference=w495, error in=w496) -> (error out=w499:errorcluster, "Controls[]"=w497:refnum<vi>[])  [unwired: 1 out]
            n233 = Index Array(array=w497, index=3) -> (element=w523:refnum<vi>)
            n234 = To More Specific Class(target class=w500, reference=w523, error in=w499) -> (specific class reference=w501:refnum<vi>, error out=w502:errorcluster)
            n235 = invoke class="VIRef" method="Make Strict Reference"(reference=w501, error in=w502, "VI Ref"=w517) -> (error out=w503:errorcluster)  [unwired: 1 in, 3 out]
            n236 = invoke class="VI" method="Save.Instrument"(reference=w504, error in=w503) -> (error out=w522:errorcluster)  [unwired: 4 in, 5 out]
            n237 = property class="VI"(reference=w526, error in=w522) -> (reference out=w518:refnum<vi>, error out=w508:errorcluster, "Panel"=w509:refnum<vi>)
            n238 = property class="Pnl"(reference=w509, error in=w508) -> (reference out=w521:refnum<vi>, error out=w511:errorcluster, "Controls[]"=w519:refnum<vi>[])
            n239 = for {
              tunnel: w519 -> [w534] mode=indexing
              tunnel: "ProcessViRef" -> [w533]
              shift-right: [w529] -> w516
              shift-left: w511 -> [w530]
              tunnel: [w528] -> w524
              stop <- w531 stop-if-true
              n240 = property class="Ctl"(reference=w534, error in=w530) -> (reference out=w528:refnum<vi>, error out=w529:errorcluster, "Label.Text"=w532:string)
              n241 = Equal?(x=w532, y=w533) -> (x = y?=w531:bool)
            }
            n242 = To More Specific Class(target class=w515, reference=w524, error in=w516) -> (specific class reference=w514:refnum<vi>, error out=w513:errorcluster)
            n243 = invoke class="VIRef" method="Make Strict Reference"(reference=w514, error in=w513, "VI Ref"=w517) -> (error out=w512:errorcluster)  [unwired: 1 in, 3 out]
            n244 = invoke class="VI" method="Save.Instrument"(reference=w518, error in=w512) -> (error out=w487:errorcluster)  [unwired: 4 in, 5 out]
            n245 = Close Reference(reference=w519, error in (no error)=w487) -> (error out=w520:errorcluster)
            n246 = Close Reference(reference=w521, error in (no error)=w520) -> ()  [unwired: 1 out]
            n247 = Close Reference(reference=w506, error in (no error)=w522) -> (error out=w507:errorcluster)
            n248 = Close Reference(reference=w505, error in (no error)=w507) -> ()  [unwired: 1 out]
          }
          frame "UpdateIcons" {
            w567 = u8 32 ("x")
            n249 = Unbundle By Name(w546) -> ("ProcessVI"=w549:refnum<vi>, "StartVI"=w548:refnum<vi>, "StopVI"=w547:refnum<vi>, "RepositoryVI"=w538:refnum<vi>, "Data.ProcessName"=w537:string, "Data.StartName"=w541:string, "Data.StopName"=w540:string)
            n250 = property class="LVClassLibrary"(reference=w550, error in=w544) -> (reference out=w555:refnum<vi>, error out=w551:errorcluster, "Member Data"=w553:refnum<vi>)
            n251 = Build Array(w549, w548, w547, w538) -> (w542:refnum<vi>[])
            n252 = call <resource>:"GDSLvIcon_AnalyseViIcon.vi"("ViRef/LvCLassRef/LvLibRef/ViPath/2D_Image"=w553, "error in (no error)"=w551) -> ("HeaderIcon"=w556:u8[][], "error out"=w552:errorcluster)  [unwired: 5 in, 11 out]
            n253 = Close Reference(reference=w553, error in (no error)=w552) -> (error out=w554:errorcluster)
            n254 = Format Into String(format string="%sRepository", w537) -> (resulting string=w536:string)  [unwired: 2 in, 1 out]
            n255 = Array Size(array=w556) -> (size(s)=w562:i32[])
            n256 = call <resource>:"GDSLvClass_ReadClassColors.vi"("Library Refnum"=w555, "error in (no error)"=w554) -> ("LvClassIconSettings"=w558:T20, "error out"=w545:errorcluster)  [unwired: 12 in, 4 out]
            n257 = Unbundle By Name(w558) -> ("Frame"=w561:u32, "Body Text"=w560:u32, "Frame thickness"=w557:u8)
            n258 = Build Array(w537, w541, w540, w536) -> (w539:string[])
            n259 = Unbundle By Name(w558) -> ("ColorProtected"=w559:u32)
            n260 = Index Array(array=w562) -> (element #1=w564:i32)  [unwired: 2 in, 1 out]
            n261 = Multiply(x=w557, y=u8 2) -> (x*y=w565:u8)
            n262 = Add(x=w564, y=w565) -> (x+y=w566:i32)
            n263 = Increment(x=w566) -> (x+1=w568:i32)
            n264 = Subtract(x=w567, y=w568) -> (x-y=w569:i32)
            n265 = Subtract(x=w567, y=w565) -> (x-y=w570:u8)
            n266 = for {
              tunnel: w570 -> [w592]
              tunnel: w569 -> [w591]
              tunnel: w561 -> [w588]
              tunnel: w560 -> [w587]
              tunnel: w559 -> [w586]
              tunnel: w557 -> [w585]
              tunnel: w556 -> [w584]
              shift-right: [w574] -> w543
              shift-left: w545 -> [w576]
              tunnel: w542 -> [w573] mode=indexing
              tunnel: w539 -> [w572] mode=indexing
              n267 = Bundle By Name(cluster=T10 {"Text"="", "Allow Only Capital Chars"=TRUE, "Compression"=enum."Auto", "Alignment"=enum."Center"} ("Text"), "Text"=w572) -> (w590:T10)
              n268 = call <resource>:"GDSLvIcon_GenerateIconText.vi"("Text"=w590, "TextPixelHeight(5-30)"=w591, "Foreground color"=w587, "Background color"=w586, "error in (no error)"=w576, "Text Pixel width(32-FrameThicknes*2))"=w592) -> ("TextOut"=w583:u8[][], "error out"=w575:errorcluster)  [unwired: 9 in, 3 out]
              n269 = call <resource>:"GDSLvIcon_CreateIconPicture.vi"("FrameColor"=w588, "FrameThickness(1)"=w585, "HeaderIconIn"=w584, "BodyIconIn"=w583, "error in (no error)"=w575) -> ("WholeIconOut"=w578:u8[][], "error out"=w581:errorcluster)  [unwired: 9 in, 4 out]
              n270 = Reshape Array(w578, 1024 ("dimension size")) -> (w580:u8[])
              n271 = Bundle By Name(cluster=T13 {"image type"=0, "image depth"=8, "image"=[], "mask"=[], "colors"=[], "Rectangle"={"left"=0, "top"=0, "right"=32, "bottom"=32}} ("image data"), "image"=w580) -> (w582:T13)
              n272 = invoke class="VI" method="VI Icon.Set from Image Data"(reference=w573, error in=w581, "ImageData"=w582) -> (error out=w574:errorcluster)  [unwired: 3 in, 5 out]
            }
          }
          frame "UpdateCreate?" {
            n273 = Unbundle By Name(w594) -> ("Data.AddInConstructor"=w597:bool)
            n274 = case shown="True" w597 {
              tunnel: w598 -> [w599 w620]
              tunnel: [w599 w619] -> w596
              tunnel: w594 -> [_ w618]
              tunnel: w593 -> [_ w614]
              frame False {
              }
              frame True {
                n275 = Unbundle By Name(w618) -> ("Application"=w607:refnum<vi>, "StartVI"=w617:refnum<vi>, "ClassProvider"=w615:T3, "TemplateName"=w604:string)
                n276 = property class="LVClassLibrary"(reference=w614) -> ("Path"=w613:path)  [unwired: 1 in, 2 out]
                n277 = To Lower Case(string=w604) -> (all lower case string=w603:string)
                n278 = Strip Path(path=w613) -> (stripped path=w612:path)  [unwired: 1 out]
                n279 = Match Pattern(string=w603, regular expression="singleton") -> (offset past match=w601:i32)  [unwired: 1 in, 3 out]
                n280 = Greater Or Equal To 0?(x=w601) -> (x >= 0?=w600:bool)
                n281 = property class="VI"(reference=w617) -> ("Path"=w616:path)  [unwired: 1 in, 2 out]
                n282 = case shown="\"EndevoGOOP3\", \"EndevoGOOP4\"" w615 {
                  tunnel: ["*Init.vi" w641 "*_Create.vi" "Constructor*.vi"] -> w611
                  tunnel: w600 -> [_ w640 _ _]
                  frame "Native", Default {
                  }
                  frame "EndevoGOOP3", "EndevoGOOP4" {
                    n283 = case shown="True" w640 {
                      tunnel: ["*Init.vi" "*_Create.vi"] -> w641
                      frame True {
                      }
                      frame False {
                      }
                    }
                  }
                  frame "OpenG(RootObject)" {
                  }
                  frame "OpenG(OpenG_Object)" {
                  }
                }
                n284 = call <vilib>:"Recursive File List.vi"("pattern"=w611, "Treat LLBs as Folders?"=TRUE, "Folder Path"=w612) -> ("All Files in Dir"=w609:path[])  [unwired: 4 in, 4 out]
                n285 = Index Array(array=w609) -> (element=w606:path)  [unwired: 1 in]
                n286 = call <vilib>:"Check if File or Folder Exists.vi"("path"=w606) -> ("file or folder exists?"=w608:bool)  [unwired: 8 in, 2 out]
                n287 = case shown="True" w608 {
                  tunnel: w620 -> [w621 w622]
                  tunnel: [w621 w623] -> w619
                  tunnel: w616 -> [_ w634]
                  tunnel: w607 -> [_ w632]
                  tunnel: w606 -> [_ w631]
                  tunnel: "The \"Start Process VI\" could not automatically be placed in the Create/Construct method.\nPlease add this method manually." ("message") -> [_ w625]
                  frame False {
                  }
                  frame True {
                    n288 = Open VI Reference(application reference (local)=w632, vi path=w631, error in (no error)=w622) -> (vi reference=w630:refnum<vi>, error out=w633:errorcluster)  [unwired: 3 in]
                    n289 = call <resource>:"Scripting_AddVIInsideNoErrorCase.vi"("ViToModify"=w630, "VIToAdd"=w634, "error in (no error)"=w633, "AddVIOnLeftSideCaseStructure"=FALSE, "OnlyReference"=FALSE) -> ("error out"=w629:errorcluster)  [unwired: 14 in]
                    n290 = invoke class="VI" method="Save.Instrument"(reference=w630, error in=w629) -> (reference out=w627:refnum<vi>, error out=w628:errorcluster)  [unwired: 4 in, 4 out]
                    n291 = Close Reference(reference=w627, error in (no error)=w628) -> (error out=w624:errorcluster)
                    n292 = case shown="Error" w624 {
                      selector: w624 -> [w636 _]
                      tunnel: [w636 w638] -> w623
                      tunnel: w622 -> [_ w638]
                      tunnel: w625 -> [_ w637]
                      frame No Error {
                      }
                      frame Error {
                        n293 = One Button Dialog(message=w637) -> ()  [unwired: 1 in, 1 out]
                      }
                    }
                  }
                }
              }
            }
          }
          frame "UpdateDestroy?" {
            n294 = Unbundle By Name(w647) -> ("Data.AddInDestructor"=w650:bool)
            n295 = case shown="True" w650 {
              tunnel: w651 -> [w652 w662]
              tunnel: [w652 w661] -> w649
              tunnel: w647 -> [_ w660]
              tunnel: w646 -> [_ w659]
              frame False {
              }
              frame True {
                n296 = Unbundle By Name(w660) -> ("Application"=w664:refnum<vi>, "StopVI"=w673:refnum<vi>, "ClassProvider"=w671:T3, "TemplateName"=w654:string)
                n297 = To Lower Case(string=w654) -> (all lower case string=w657:string)
                n298 = property class="LVClassLibrary"(reference=w659) -> ("Path"=w670:path)  [unwired: 1 in, 2 out]
                n299 = Strip Path(path=w670) -> (stripped path=w669:path)  [unwired: 1 out]
                n300 = Match Pattern(string=w657, regular expression="singleton") -> (offset past match=w655:i32)  [unwired: 1 in, 3 out]
                n301 = Greater Or Equal To 0?(x=w655) -> (x >= 0?=w653:bool)
                n302 = case shown="\"EndevoGOOP3\", \"EndevoGOOP4\"" w671 {
                  tunnel: ["CleanUp.vi" w705 "Destroy.vi" "Destructor*.vi"] -> w668
                  tunnel: w653 -> [_ w704 _ _]
                  frame "Native", Default {
                  }
                  frame "EndevoGOOP3", "EndevoGOOP4" {
                    n303 = case shown="True" w704 {
                      tunnel: ["*CleanUp.vi" "Destroy.vi"] -> w705
                      frame True {
                      }
                      frame False {
                      }
                    }
                  }
                  frame "OpenG(RootObject)" {
                  }
                  frame "OpenG(OpenG_Object)" {
                  }
                }
                n304 = call <vilib>:"Recursive File List.vi"("pattern"=w668, "Treat LLBs as Folders?"=TRUE, "Folder Path"=w669) -> ("All Files in Dir"=w666:path[])  [unwired: 4 in, 4 out]
                n305 = property class="VI"(reference=w673) -> ("Path"=w672:path)  [unwired: 1 in, 2 out]
                n306 = Index Array(array=w666) -> (element=w663:path)  [unwired: 1 in]
                n307 = call <vilib>:"Check if File or Folder Exists.vi"("path"=w663) -> ("file or folder exists?"=w665:bool)  [unwired: 8 in, 2 out]
                n308 = case shown="True" w665 {
                  tunnel: w662 -> [w674 w677]
                  tunnel: [w674 w678] -> w661
                  tunnel: w672 -> [_ w687]
                  tunnel: w664 -> [_ w685]
                  tunnel: w663 -> [_ w684]
                  tunnel: "The \"Stop Process VI\" could not automatically be placed in the Destroy/Destruct method.\nPlease add this method manually before the object is destroyed." ("message") -> [_ w676]
                  tunnel: w653 -> [_ w675]
                  frame False {
                  }
                  frame True {
                    n309 = Open VI Reference(application reference (local)=w685, vi path=w684, error in (no error)=w677) -> (vi reference=w683:refnum<vi>, error out=w686:errorcluster)  [unwired: 3 in]
                    n310 = case shown="True" w675 {
                      tunnel: w687 -> [w692 w699]
                      tunnel: w686 -> [w691 w698]
                      tunnel: w683 -> [w690 w696]
                      tunnel: [w689 w697] -> w682
                      frame False {
                        n311 = call <resource>:"Scripting_AddVIInsideNoErrorCase.vi"("ViToModify"=w690, "VIToAdd"=w692, "error in (no error)"=w691, "AddVIOnLeftSideCaseStructure"=TRUE, "OnlyReference"=TRUE) -> ("error out"=w689:errorcluster)  [unwired: 14 in]
                      }
                      frame True {
                        n312 = call <resource>:"Scripting_AddVIBetweenVIs.vi"("ViToModify"=w696, "VIToAdd"=w699, "VIOne(Path,Name or NamePattern)"="GetInstance.vi" ("regular expression"), "VITwo(Path,Name or NamePattern), If Left/Right-string, it will be placed to the right or left of VIOne"="GetAttributes.vi" ("regular expression"), "error in (no error)"=w698) -> ("error out"=w697:errorcluster)  [unwired: 13 in, 1 out]
                      }
                    }
                    n313 = invoke class="VI" method="Save.Instrument"(reference=w683, error in=w682) -> (reference out=w680:refnum<vi>, error out=w681:errorcluster)  [unwired: 4 in, 4 out]
                    n314 = Close Reference(reference=w680, error in (no error)=w681) -> (error out=w679:errorcluster)
                    n315 = case shown="Error" w679 {
                      selector: w679 -> [w700 _]
                      tunnel: [w700 w702] -> w678
                      tunnel: w677 -> [_ w702]
                      tunnel: w676 -> [_ w701]
                      frame No Error {
                      }
                      frame Error {
                        n316 = One Button Dialog(message=w701) -> ()  [unwired: 1 in, 1 out]
                      }
                    }
                  }
                }
              }
            }
          }
          frame "SaveAll" {
            n317 = Unbundle By Name(w712) -> ("ProcessVI"=w713:refnum<vi>, "Data.ProcessCreation"=w714:T1)
            n318 = case shown="\"Create only one process for this class\"" w714 {
              tunnel: w713 -> [_ w723]
              tunnel: w710 -> [w719 w721]
              tunnel: [w719 w720] -> w711
              frame "Create one process per object instance", Default {
              }
              frame "Create only one process for this class" {
                n319 = property class="VI"(reference=w723, error in=w721, "Exec.IsReentrant"=FALSE ("Execution:Is Reentrant")) -> (error out=w720:errorcluster)  [unwired: 1 out]
              }
            }
            n320 = call <resource>:"GDSLvClass_SaveEverythingInClass.vi"("ClassRefIn"=w716, "ForceResaving(False)"=TRUE, "error in"=w711) -> ("error out"=w717:errorcluster)  [unwired: 15 in, 1 out]
          }
        }
        n321 = Equal?(x=w153, y="Exit") -> (x = y?=w156:bool)
        n322 = Select(t="Error", s=w152, f=w153) -> (s? t:f=w157:string)
      }
    }
    frame "RemovePattern" {
    }
    frame "UpdatePattern" {
    }
    frame "CreatePatternMethod" {
      w732 = "Init"
      n323 = property class="VI"(error in=w731, "Front Panel.Open"=FALSE ("Front Panel Window:Open")) -> (error out=w733:errorcluster)  [unwired: 1 in, 1 out]
      n324 = while {
        shift-right: [w742] -> w726
        shift-left: w733 -> [w749]
        shift-right: [w747] -> _
        shift-left: w732 -> [w748]
        shift-right: [w735] -> _
        shift-left: _ -> [w741]
        tunnel: w729 -> [w740]
        tunnel: w727 -> [w739]
        tunnel: w728 -> [w738]
        tunnel: w730 -> [w737]
        shift-left: w732 -> [w736]
        stop <- w746 stop-if-true
        n325 = case shown="\"Init\"" w748 {
          tunnel: w749 -> [w778 w796 w818]
          tunnel: [w770 w795 w819] -> w742
          tunnel: [w768 "ReplaceProcessRepositoryVI" "Exit"] -> w743
          tunnel: w741 -> [_ w782 w821]
          tunnel: w740 -> [w779 _ _]
          tunnel: w739 -> [_ _ _]
          tunnel: w738 -> [w759 _ _]
          tunnel: w737 -> [w771 w797 w820]
          tunnel: w736 -> [_ _ _]
          tunnel: [w753 w782 w821] -> w735
          frame "Init" {
            n326 = Variant To Data(error in=w778, type=cluster{path, "VI":refnum<vi>, "Name":string} {path "", "VI"=refnum, "Name"=""} ("cluster"), Variant=w779) -> (data=w761:cluster{path, "VI":refnum<vi>, "Name":string}, error out=w763:errorcluster)
            n327 = Unbundle(w761) -> (w758:path, "VI"=w757:refnum<vi>, "Name"=w750:string)
            n328 = call <resource>:"GDSLvClass_ReadClassType.vi"("Class Refnum In"=w771, "error in (no error)"=w763) -> ("ClassSettings"=w777:T14, "error out"=w770:errorcluster)  [unwired: 15 in, 1 out]
            n329 = Unbundle By Name(w777) -> ("ConnectorPanePattern"=w776:string, "ClassTemplateUsed"=w775:string)
            n330 = To Lower Case(string=w775) -> (all lower case string=w773:string)
            n331 = case shown="\"0\", Default" w776 {
              tunnel: ["4x4x4" "6x8x6"] -> _
              frame "0", Default {
              }
              frame "1", "2" {
              }
            }
            n332 = Match Pattern(string=w773, regular expression="singleton" ("search string")) -> (offset past match=w774:i32)  [unwired: 1 in, 3 out]
            n333 = Greater Or Equal To 0?(x=w774) -> (x >= 0?=w769:bool)
            n334 = Current VI's Path() -> (path=w766:path)
            n335 = Strip Path(path=w766) -> (stripped path=w765:path)  [unwired: 1 out]
            n336 = Build Path(base path=w765, name or relative path="ActiveObjects_QueueQueue_SubVIs") -> (appended path=w756:path)
            n337 = Build Path(base path=w756, name or relative path="ActiveObject_QueueQueue_ProcessRepository_Native.vi") -> (appended path=w754:path)
            n338 = Build Path(base path=w756, name or relative path="ActiveObject_QueueQueue_Process.vi") -> (appended path=w751:path)
            n339 = Bundle By Name(cluster=w759, "MethodTemplate"=w758, "VI"=w757, "SupportFolder"=w756, "VI_ToFind"=w754, "VI_ToFindSingleton"=w751, "Name"=w750) -> (w753:T4)
            n340 = Select(t="Place_GetInstanceVI", s=w769, f="ReplaceProcessRepositoryVI") -> (s? t:f=w768:string)
          }
          frame "Place_GetInstanceVI" {
            n341 = call <resource>:"GDSLvClass_GetClassMethod.vi"("Class Refnum In"=w797, "VINames"=string[] ["GetInstance.vi$"] ("VIsToSerachFor/ViName"), "error in (no error)"=w796) -> ("ViPaths"=w793:path[], "error out"=w788:errorcluster)  [unwired: 13 in, 2 out]
            n342 = Unbundle By Name(w782) -> ("VI_ToFindSingleton"=w787:path, "VI"=w783:refnum<vi>)
            n343 = Build Array(w787) -> (w786:path[])
            n344 = call <resource>:"Scripting_FindVisOnDiagram.vi"("ViRef"=w783, "VIsToSerachFor/ViName"=w786, "error in (no error)"=w788) -> ("VisFound"=w790:refnum<vi>[], "error out"=w789:errorcluster)  [unwired: 15 in]
            n345 = Index Array(array=w793) -> (element=w785:path)  [unwired: 1 in]
            n346 = Index Array(array=w790) -> (element=w791:refnum<vi>)  [unwired: 1 in]
            n347 = invoke class="GObj" method="Replace"(reference=w791, error in=w789, "Path"=w785) -> (error out=w784:errorcluster, "Replace"=w792:refnum<vi>)  [unwired: 3 in, 4 out]
            n348 = Close Reference(reference=w790, error in (no error)=w784) -> ()  [unwired: 1 out]
            n349 = Close Reference(reference=w792, error in (no error)=w784) -> (error out=w795:errorcluster)
          }
          frame "ReplaceGetClassAttributes", Default {
            w805 = "Repository.vi$"
            n350 = Unbundle By Name(w821) -> ("VI_ToFind"=w811:path, "VI"=w807:refnum<vi>, "Name"=w806:string)
            n351 = Build Array(w811) -> (w810:path[])
            n352 = Concatenate Strings(w806, w805) -> (w804:string)
            n353 = Build Array(w804, w805) -> (w799:string[])
            n354 = call <resource>:"GDSLvClass_GetClassMethod.vi"("Class Refnum In"=w820, "VINames"=w799, "error in (no error)"=w818) -> ("ViPaths"=w808:path[], "error out"=w809:errorcluster)  [unwired: 13 in, 2 out]
            n355 = Index Array(array=w808) -> (element #1=w801:path, element #2=w802:path)  [unwired: 2 in]
            n356 = Empty String/Path?(string/path=w801) -> (empty?=w803:bool)
            n357 = Select(t=w802, s=w803, f=w801) -> (s? t:f=w800:path)
            n358 = call <resource>:"Scripting_FindVisOnDiagram.vi"("ViRef"=w807, "VIsToSerachFor/ViName"=w810, "error in (no error)"=w809) -> ("VisFound"=w814:refnum<vi>[], "error out"=w813:errorcluster)  [unwired: 15 in]
            n359 = Index Array(array=w814) -> (element=w816:refnum<vi>)  [unwired: 1 in]
            n360 = invoke class="GObj" method="Replace"(reference=w816, error in=w813, "Path"=w800) -> (error out=w817:errorcluster, "Replace"=w815:refnum<vi>)  [unwired: 3 in, 4 out]
            n361 = Close Reference(reference=w814, error in (no error)=w817) -> ()  [unwired: 1 out]
            n362 = Close Reference(reference=w815, error in (no error)=w817) -> (error out=w812:errorcluster)
            n363 = invoke class="VI" method="Save.Instrument"(reference=w807, error in=w812) -> (error out=w819:errorcluster)  [unwired: 4 in, 5 out]
          }
        }
        n364 = Equal?(x=w743, y="Exit") -> (x = y?=w746:bool)
        n365 = Select(t="Error", s=w742, f=w743) -> (s? t:f=w747:string)
      }
    }
  }
  "error out" <- w8
  "DataOut" <- w5
  "Cancelled" <- w6
  "Name" <- w1
